vi "Build All of Type.vi"(8 "error in (no error)":errorcluster, 10 "Type":string="Packed Library", 11 "Path to project":path) -> (0 "error out":errorcluster)   [LabVIEW 2021]
uses:
  <vilib>/AppBuilder/AB_API_Simple/Build (path).vi
  <vilib>/AppBuilder/AB_API_Simple/NI_App_Builder_API.lvlib
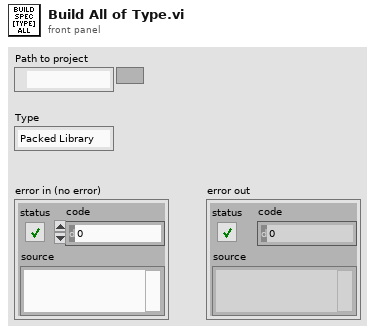
[diagram p1: front panel]
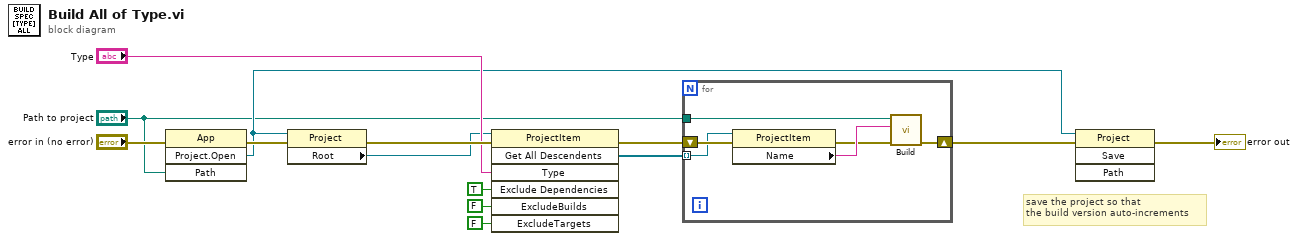
[diagram p0: block diagram]
diagram:
  # "save the project so that\nthe build version auto-increments"
  n1 = invoke class="App" method="Project.Open"(error in="error in (no error)", "Path"="Path to project") -> (error out=w6:errorcluster, "Project:Open"=w4:refnum<vi>)  [unwired: 2 in, 2 out]
  n2 = property class="Project"(reference=w4, error in=w6) -> (error out=w12:errorcluster, "Root"=w7:refnum<vi>)  [unwired: 1 out]
  n3 = invoke class="ProjectItem" method="Get All Descendents"(reference=w7, error in=w12, "Type"="Type", "Exclude Dependencies"=TRUE ("ExcludeDependencies"), "ExcludeBuilds"=FALSE, "ExcludeTargets"=FALSE) -> (error out=w13:errorcluster, "All Descendents"=w1:refnum<vi>[])  [unwired: 1 in, 5 out]
  n4 = for {
    tunnel: "Path to project" -> [w16]
    shift-right: [w17] -> w5
    shift-left: w13 -> [w18]
    tunnel: w1 -> [w15] mode=indexing
    n5 = property class="ProjectItem"(reference=w15, error in=w18) -> (error out=w19:errorcluster, "Name"=w20:string)  [unwired: 1 out]
    n6 = call-poly <vilib>:"Build.vi"("error in (no error)"=w19, "Name of build specification (if empty: build all)"=w20, "Path to project"=w16) -> ("error out"=w17:errorcluster)  [unwired: 7 in, 1 out]
  }
  n7 = invoke class="Project" method="Save"(reference=w4, error in=w5) -> (error out=→"error out":errorcluster)  [unwired: 2 in, 3 out]
